vi "Configure Loop Setup Parameters.vi"(0 "VISA resource name":refnum<visa-resource-name>, 1 "Unit Address (1)":u8=1 min=1 max=254, 5 "Channel 1 Control Algorithm (0: Off)":u8(ring) items=["Off", "On/Off", "PID", "MTR"], 7 "Channel 2 Control Algorithm (0: Off)":u8(ring) items=["Off", "On/Off", "PID"], 9 "Control Action (0: Reverse)":u16(ring) items=["Reverse", "Direct"], 11 "error in (no error)":errorcluster) -> (4 "VISA resource name out":refnum<visa-resource-name>, 15 "error out":errorcluster)   [LabVIEW 2010, in "Eurotherm 32xx Series.lvlib"]
doc: "This VI configures Loop Setup parameters.\n\nDescription:\n\nOn/Off Control -\nOn/Off control is the simplest means of control but gives rise to fluctuations in the process variable. A degree of hysteresis or deadband must be set in On/Off control if the operation of the switching device is to be reduced and relay chatter is to be avoided.\nOn/Off control is a very simple form of control, which leads to oscillation of the process variable. This oscillation can affect the quality of the final product and is undesirable. The alternative is to use three term control, known as PID control.\n\nPID Control -\nPID or Three Term Control is an algorithm which controls the process to a setpoint. PID provides more stable control by continuously adjusting the output to compensate for the Error, the rate of change or the error and any continuous offsets.\nPID controllers must be tuned to the process they are controlling-\n-A too small proportional band gives temperature cycling (control loop instability). \n-A too large proportional band gives sluggish control, (a too feeble change of power in response to deviations of temperature). \n-A too small integral time will give an over eager response and result in instability. \n-A too large integral time will slow down both the approach to set point on a start up and return to set point after a disturbance. \n-Although derivative action helps to achieve stability a too large derivative time can also bring instability by an over eager power boost or throttle back. \n\nMotorised Valve Control-\nThe controller may be configured for motorised valve control as an alternative to the standard PID control algorithm. This algorithm is designed specifically for positioning motorised valves.\nThe control is performed by delivering open or close pulses in response to the control demand signal.\nThe motorised valve algorithm operates in boundless mode, which does not require a position feedback potentiometer for control purposes; although one can be connected and used purely to display the valve’s position. \n\nWarning: This VI uses Controller Configuration Mode, this interrupts working process (device will not control).\nIt is recommended that the device should be disconnected from any active process."
uses:
  <instrlib>/Eurotherm 32xx Series/Eurotherm 32xx Series.lvlib
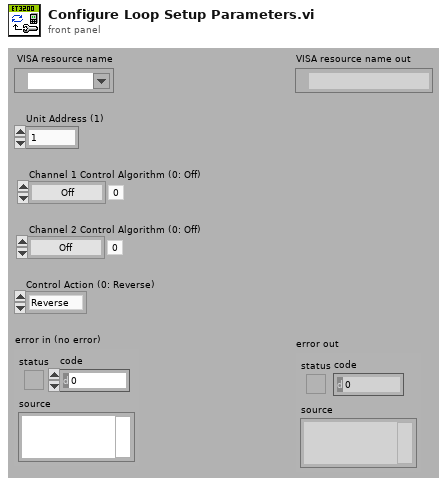
[diagram p1: front panel]
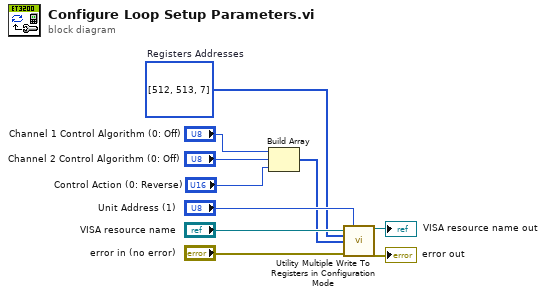
[diagram p0: block diagram]
diagram:
  w3 = u16[] [512, 513, 7]  # Registers Addresses
  n1 = Build Array("Channel 1 Control Algorithm (0: Off)", "Channel 2 Control Algorithm (0: Off)", "Control Action (0: Reverse)") -> (w2:u16[])
  n2 = call <instrlib>:"Utility Multiple Write To Registers in Configuration Mode.vi"("VISA resource name"="VISA resource name", "Unit Address (1)"="Unit Address (1)", "Registers Addresses (0)"=w3, "Data (0)"=w2, "error in (no error)"="error in (no error)") -> ("VISA resource name out"=→"VISA resource name out":refnum<visa-resource-name>, "error out"=→"error out":errorcluster)  [unwired: 9 in]
